vi "Revision Query.vi"(8 "error in (no error)":errorcluster, 11 "VISA resource name":refnum<visa-resource-name>) -> (0 "error out":errorcluster, 1 "instr firmware revision":string, 2 "instr driver revision":string, 3 "VISA resource name out":refnum<visa-resource-name>)   [LabVIEW 2013]
doc: "This VI queries the current instrument firmware revision and instrument driver revision.\n\nAgilent Technologies E364xA Series DC Power Supply\nCreated By: MVV National Instruments\nRelease Date: April 2003\nVersion: 1.11\nOriginally Developed in LabVIEW Version: 7.0\n\nModification History: \n\n6//11/03\n- Fixed serial communications control to work properly\n- Removed unnecessary utility age364xa write VI\n- Fixed Measurement VI to measure actual value and not programmed value.\n\n6/13/03\n- Fixed Serial I/O Flush Buffer Size\n\nNone"
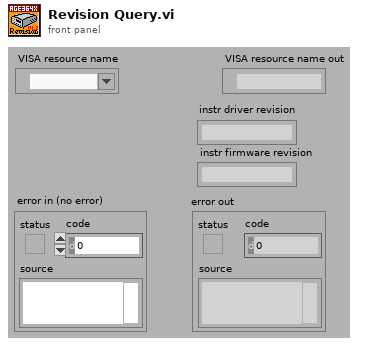
[diagram p1: front panel]
types:
  T1 = enum32{"invalid app kind", "Development System", "Run Time System", "Student Edition", "Embedded LabVIEW", "Evaluation", "Custom"}
  T2 = cluster{"Major":u16, "Minor":u16, "Fix":u16, "Build":u16}
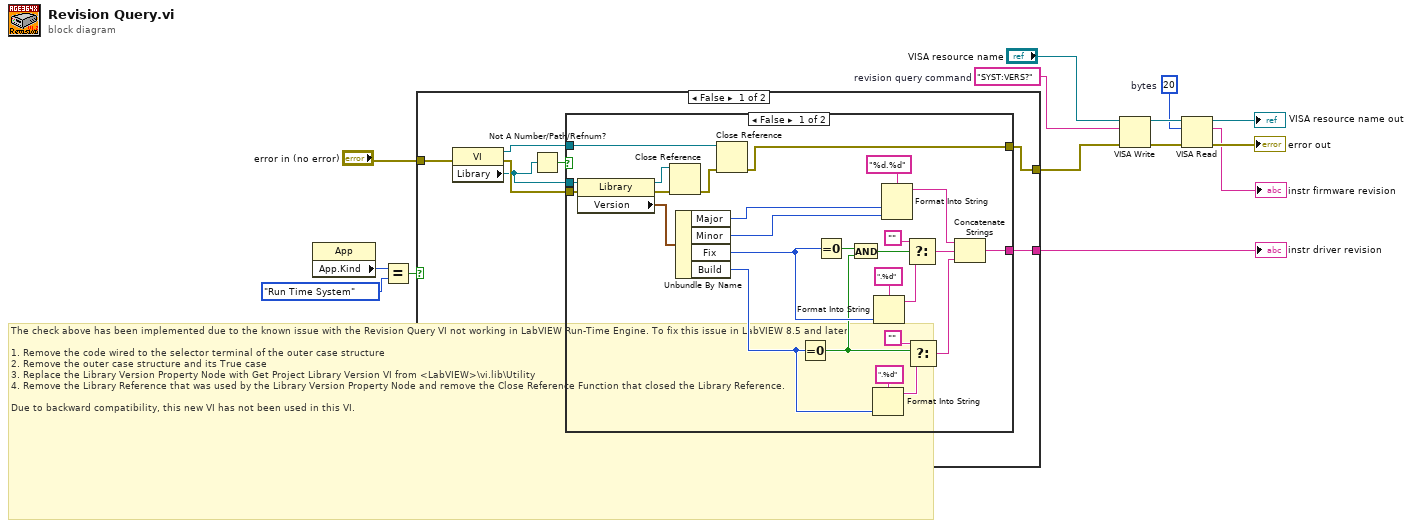
[diagram p0: block diagram]
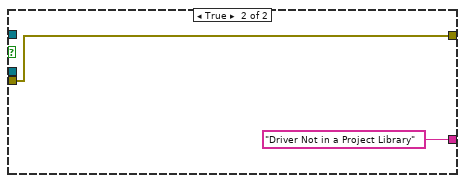
[diagram p2: hidden frame]
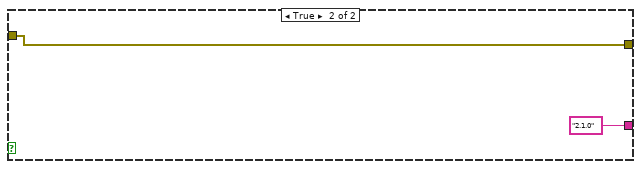
[diagram p3: hidden frame]
diagram:
  w7 = u32 20  # bytes
  w14 = "SYST:VERS?"  # revision query command
  # "The check above has been implemented due to the known issue with the Revision Query VI not working in LabVIEW Run-Time Engine. To fix this issue in LabVIEW 8.5 and later:\n\n1. Remove the code wired to the selector terminal of the outer case structure\n2. Remove the outer case structure and its True case\n3. Replace the Library Version Property Node with Get Project Library Version VI from <LabVIEW>\\vi.lib\\Utility\n4. Remove the Library Reference that was used by the Library Version Property Node and remove the Close Reference Function that closed the Library Reference.\n\nDue to backward compatibility, this new VI has not been used in this VI."
  n1 = property class="App"() -> ("App.Kind"=w2:T1)  [unwired: 2 in, 2 out]
  n2 = Equal?(x=w2, y=T1."Run Time System") -> (x = y?=w3:bool)
  n3 = case shown="False" w3 {
    tunnel: "error in (no error)" -> [w21 w51]
    tunnel: [w16 "2.1.0"] -> w5
    tunnel: [w15 w51] -> w4
    frame False {
      n4 = property class="VI"(error in=w21) -> (reference out=w17:refnum<vi>, error out=w20:errorcluster, "Library"=w19:refnum<vi>)  [unwired: 1 in]
      n5 = Not A Number/Path/Refnum?(number/path/refnum=w19) -> (NaN/Path/Refnum?=w18:bool)
      n6 = case shown="False" w18 {
        tunnel: [w26 w48] -> w15
        tunnel: [w25 "Driver Not in a Project Library"] -> w16
        tunnel: w20 -> [w24 w48]
        tunnel: w19 -> [w23 _]
        tunnel: w17 -> [w22 _]
        frame False {
          n7 = property class="Library"(reference=w23, error in=w24) -> (reference out=w46:refnum<vi>, error out=w47:errorcluster, "Version"=w44:T2)
          n8 = Close Reference(reference=w46, error in (no error)=w47) -> (error out=w45:errorcluster)
          n9 = Unbundle By Name(w44) -> ("Major"=w33:u16, "Minor"=w32:u16, "Fix"=w30:u16, "Build"=w31:u16)
          n10 = Close Reference(reference=w22, error in (no error)=w45) -> (error out=w26:errorcluster)
          n11 = Equal To 0?(x=w31) -> (x = 0?=w28:bool)
          n12 = Equal To 0?(x=w30) -> (x = 0?=w29:bool)
          n13 = And(x=w29, y=w28) -> (x .and. y?=w27:bool)
          n14 = Format Into String(format string=".%d", w31) -> (resulting string=w37:string)  [unwired: 2 in, 1 out]
          n15 = Format Into String(format string=".%d", w30) -> (resulting string=w41:string)  [unwired: 2 in, 1 out]
          n16 = Format Into String(format string="%d.%d", w33, w32) -> (resulting string=w39:string)  [unwired: 2 in, 1 out]
          n17 = Select(t="", s=w27, f=w41) -> (s? t:f=w38:string)
          n18 = Select(t="", s=w28, f=w37) -> (s? t:f=w34:string)
          n19 = Concatenate Strings(w39, w38, w34) -> (w25:string)
        }
        frame True {
        }
      }
    }
    frame True {
    }
  }
  "instr driver revision" <- w5
  n20 = VISA Write(VISA resource name="VISA resource name", write buffer=w14, error in (no error)=w4) -> (VISA resource name out=w8:refnum<visa-resource-name>, error out=w11:errorcluster)  [unwired: 1 out]
  n21 = VISA Read(VISA resource name=w8, byte count=w7, error in (no error)=w11) -> (VISA resource name out=→"VISA resource name out":refnum<visa-resource-name>, read buffer=→"instr firmware revision":string, error out=→"error out":errorcluster)  [unwired: 1 out]
